vi "LocalVariables.vi"() -> ()   [LabVIEW 2014]
panel:
  out "Flash Period (ms)":u32
  in  "Flash Frequency (Hz)":dbl=0.5
  in  "stop":bool
  out "Bool at Program Start":bool
  in  "My Bool":bool
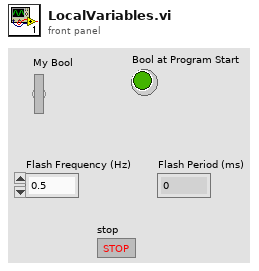
[diagram p1: front panel]
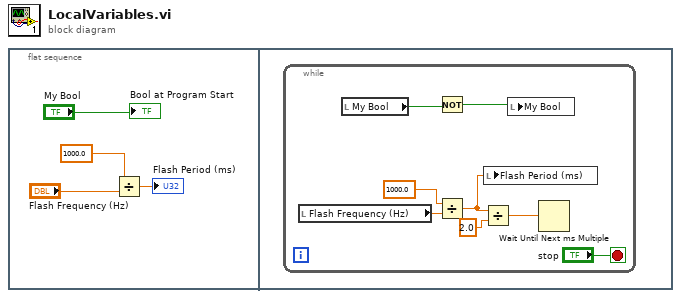
[diagram p0: block diagram]
diagram:
  n1 = flat-sequence {
    frame #0 {
      n2 = Divide(x=1000.0, y="Flash Frequency (Hz)") -> (x/y=→"Flash Period (ms)":dbl)
      "Bool at Program Start" <- "My Bool"
    }
    frame #1 {
      n3 = while {
        stop <- "stop" stop-if-true
        n4 = local read "Flash Frequency (Hz)"() -> (w9:dbl)
        n5 = local read "My Bool"() -> (w11:bool)
        n6 = Not(x=w11) -> (.not. x?=w10:bool)
        n7 = Divide(x=1000.0, y=w9) -> (x/y=w7:dbl)
        n8 = Divide(x=w7, y=2.0) -> (x/y=w5:dbl)
        n9 = local write "Flash Period (ms)"(w7) -> ()
        n10 = local write "My Bool"(w10) -> ()
        n11 = Wait Until Next ms Multiple(millisecond multiple=w5) -> ()  [unwired: 1 out]
      }
    }
  }
